vi "Draw.vi"(8 "error in (no error)":errorcluster, 10 "Picture in":picture, 11 "Triangle in":refnum<class "Rectangle.lvclass">) -> (0 "error out":errorcluster, 2 "Picture out":picture, 3 "Triangle out":refnum<class "Rectangle.lvclass">)   [LabVIEW 2015, in "Rectangle.lvclass"]
uses:
  Rectangle.lvclass
  Graphic/Graphic.lvclass/Graphic.ctl
  Line/Line.lvclass
  Polygon/Polygon.lvclass/Polygon.ctl
  Polygon/Polygon.lvclass
  Graphic/Graphic.lvclass
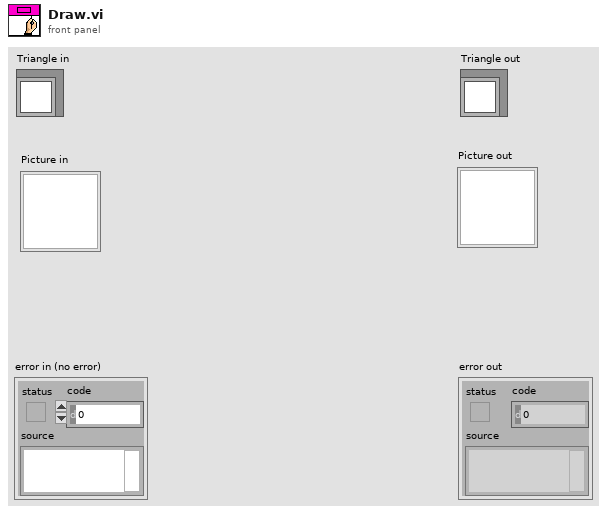
[diagram p1: front panel]
types:
  T1 = typedef "Graphic.lvclass/Style.ctl" = cluster{"Color":u32, "Pen":cluster{"Width":u16, "Style":enum32{"Solid", "Dash", "Dot", "DashDot", "DashDotDot"}}}
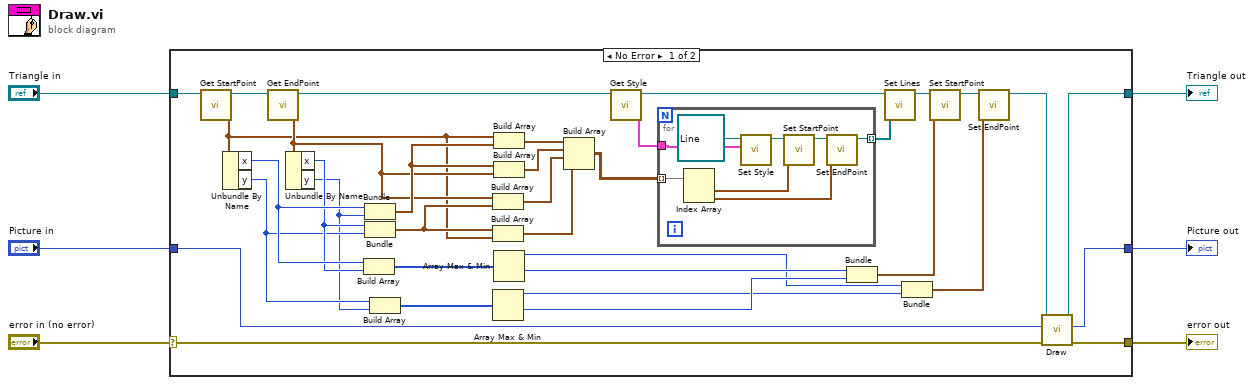
[diagram p0: block diagram]
diagram:
  n1 = case shown="No Error" "error in (no error)" {
    selector: "error in (no error)" -> [w38 w52]
    tunnel: [w41 w52] -> w6
    tunnel: [w40 w50] -> w5
    tunnel: [w39 w51] -> w4
    tunnel: "Picture in" -> [w37 w50]
    tunnel: "Triangle in" -> [w36 w51]
    frame No Error {
      n2 = call "Get StartPoint.vi"("Graphic in"=w36) -> ("StartPoint"=w25:cluster{"x":i16, "y":i16}, "Graphic out"=w35:refnum<class "Rectangle.lvclass">)  [unwired: 8 in, 1 out]
      n3 = Unbundle By Name(w25) -> ("x"=w23:i16, "y"=w21:i16)
      n4 = call "Get EndPoint.vi"("Graphic in"=w35) -> ("EndPoint"=w27:cluster{"x":i16, "y":i16}, "Graphic out"=w34:refnum<class "Rectangle.lvclass">)  [unwired: 8 in, 1 out]
      n5 = Unbundle By Name(w27) -> ("x"=w22:i16, "y"=w20:i16)
      n6 = Build Array(w23, w22) -> (w19:i16[])
      n7 = Bundle("x"=w23, "y"=w20) -> (w28:cluster{"x":i16, "y":i16})  [unwired: 1 in]
      n8 = Bundle("x"=w22, "y"=w21) -> (w26:cluster{"x":i16, "y":i16})  [unwired: 1 in]
      n9 = Build Array(w21, w20) -> (w18:i16[])
      n10 = Build Array(w27, w26) -> (w31:cluster{"x":i16, "y":i16}[])
      n11 = Build Array(w26, w25) -> (w24:cluster{"x":i16, "y":i16}[])
      n12 = Array Max & Min(array=w18) -> (max value=w11:i16, min value=w13:i16)  [unwired: 2 out]
      n13 = Build Array(w25, w28) -> (w33:cluster{"x":i16, "y":i16}[])
      n14 = Build Array(w28, w27) -> (w32:cluster{"x":i16, "y":i16}[])
      n15 = Array Max & Min(array=w19) -> (max value=w12:i16, min value=w14:i16)  [unwired: 2 out]
      n16 = Build Array(w33, w32, w31, w24) -> (w30:cluster{"x":i16, "y":i16}[][])
      n17 = call "Get Style.vi"("Graphic in"=w34) -> ("Style"=w7:T1, "Graphic out"=w8:refnum<class "Rectangle.lvclass">)  [unwired: 8 in, 1 out]
      n18 = for {
        tunnel: w30 -> [w47] mode=indexing
        tunnel: [w44] -> w29 mode=indexing
        tunnel: w7 -> [w42]
        n19 = Index Array(array=w47) -> (element #1=w46:cluster{"x":i16, "y":i16}, element #2=w45:cluster{"x":i16, "y":i16})  [unwired: 2 in]
        n20 = call "Set Style.vi"("Style"=w42, "Graphic in"=refnum<class "Line.lvclass"> refnum ("Line.lvclass")) -> ("Graphic out"=w43:refnum<class "Line.lvclass">)  [unwired: 8 in, 1 out]
        n21 = call "Set StartPoint.vi"("StartPoint"=w46, "Graphic in"=w43) -> ("Graphic out"=w48:refnum<class "Line.lvclass">)  [unwired: 8 in, 1 out]
        n22 = call "Set EndPoint.vi"("EndPoint"=w45, "Graphic in"=w48) -> ("Graphic out"=w44:refnum<class "Line.lvclass">)  [unwired: 8 in, 1 out]
      }
      n23 = Bundle(w14, w13) -> (w10:cluster{i16, i16})  [unwired: 1 in]
      n24 = call "Set Lines.vi"("Lines"=w29, "Polygon in"=w8) -> ("Polygon out"=w16:refnum<class "Rectangle.lvclass">)  [unwired: 8 in, 1 out]
      n25 = Bundle(w12, w11) -> (w9:cluster{i16, i16})  [unwired: 1 in]
      n26 = call "Set StartPoint.vi"("StartPoint"=w10, "Graphic in"=w16) -> ("Graphic out"=w17:refnum<class "Rectangle.lvclass">)  [unwired: 8 in, 1 out]
      n27 = call "Set EndPoint.vi"("EndPoint"=w9, "Graphic in"=w17) -> ("Graphic out"=w15:refnum<class "Rectangle.lvclass">)  [unwired: 8 in, 1 out]
      n28 = call-parent "Draw.vi"("error in (no error)"=w38, "Picture in"=w37, "Polygon in"=w15) -> ("error out"=w41:errorcluster, "Picture out"=w40:picture, "Polygon out"=w39:refnum<class "Rectangle.lvclass">)  [unwired: 6 in]
    }
    frame Error {
    }
  }
  "error out" <- w6
  "Triangle out" <- w4
  "Picture out" <- w5
